vi "Ver 1.vi"() -> ()   [LabVIEW 2016]
doc: "This example VI shows how to use thermocouples to take a temperature measurement.\n\nNote:\nFor front panel measurements, make sure the Input switch is in the out position(F)\nFor plug-in card measurements, make sure the Input switch is in the in poisition(R)"
uses:
  Documents/keithley_27xx/Keithley 27XX/Public/Configure/Measurement Specific/Configure FRTD.vi
  Documents/keithley_27xx/Keithley 27XX/Public/Configure/Measurement Specific/Configure Thermocouple.vi
  Documents/keithley_27xx/Keithley 27XX/Public/Configure/Measurement Specific/Configure Thermistor.vi
  Documents/keithley_27xx/Keithley 27XX/Public/Data/Read Multiple Direct.vi
  Documents/keithley_27xx/Keithley 27XX/Keithley 27XX.lvlib
  Documents/keithley_27xx/Keithley 27XX/Public/Close.vi
panel:
  in  "Sample Size":dbl
  in  "Sensor Type":string(combo)
  in  "Delta3":dbl=1.0
  in  "Beta3":dbl=0.1
  in  "Alpha3":dbl=0.0038
  in  "Delta2":dbl=1.0
  in  "Beta2":dbl=0.1
  in  "Alpha2":dbl=0.0038
  in  "Delta1":dbl=1.0
  in  "Beta1":dbl=0.1
  in  "Alpha1":dbl=0.0038
  in  "Serial Configuration":T1={"Baud Rate (9600)"=9600, "Flow Control (1: XON/XOFF)"=1, "Termination Char (0:CR)"=0} {"Termination Char (0:CR)" items=["CR", "LF", "CRLF (Do not use)", "LFCR (Do not use)"]; "Flow Control (1: XON/XOFF)" items=["None", "XON/XOFF", "RTS/CTS (2701 Only)", "XON/XOFF & RTS/CTS (2701 Only)"]; "Baud Rate (9600)" items=["300"=300, "600"=600, "1200"=1200, "2400"=2400, "4800"=4800, "9600"=9600, "19.2k"=19200, "38.4k (2701 Only)"=38400, "57.6k (2701 Only)"=57600, "115.2k (2701 Only)"=115200]}
  in  "VISA resource name":refnum<visa-resource-name>="TCPIP0::192.168.69.200::1394::SOCKET"
  out "Output3":dbl[](array[numeric])
  in  "Channel (101) 3":string="117"
  out "Output2":dbl[](array[numeric])
  in  "Channel (101) 2":string="114"
  in  "stop":bool
  out "Output1":dbl[](array[numeric])
  in  "Channel (101)":string="113"
  in  "Temperature (0: Celsius)":u16(ring) items=["Celsius", "Fahrenheit", "Kelvin"]
  # "*For front panel measurements, make sure the Input switch is in the out position(F)*\n  For plug-in card measurements, make sure the Input switch is in the in position(R)"
  # "© 2005 National Instruments Corporation.  ALL RIGHTS RESERVED."
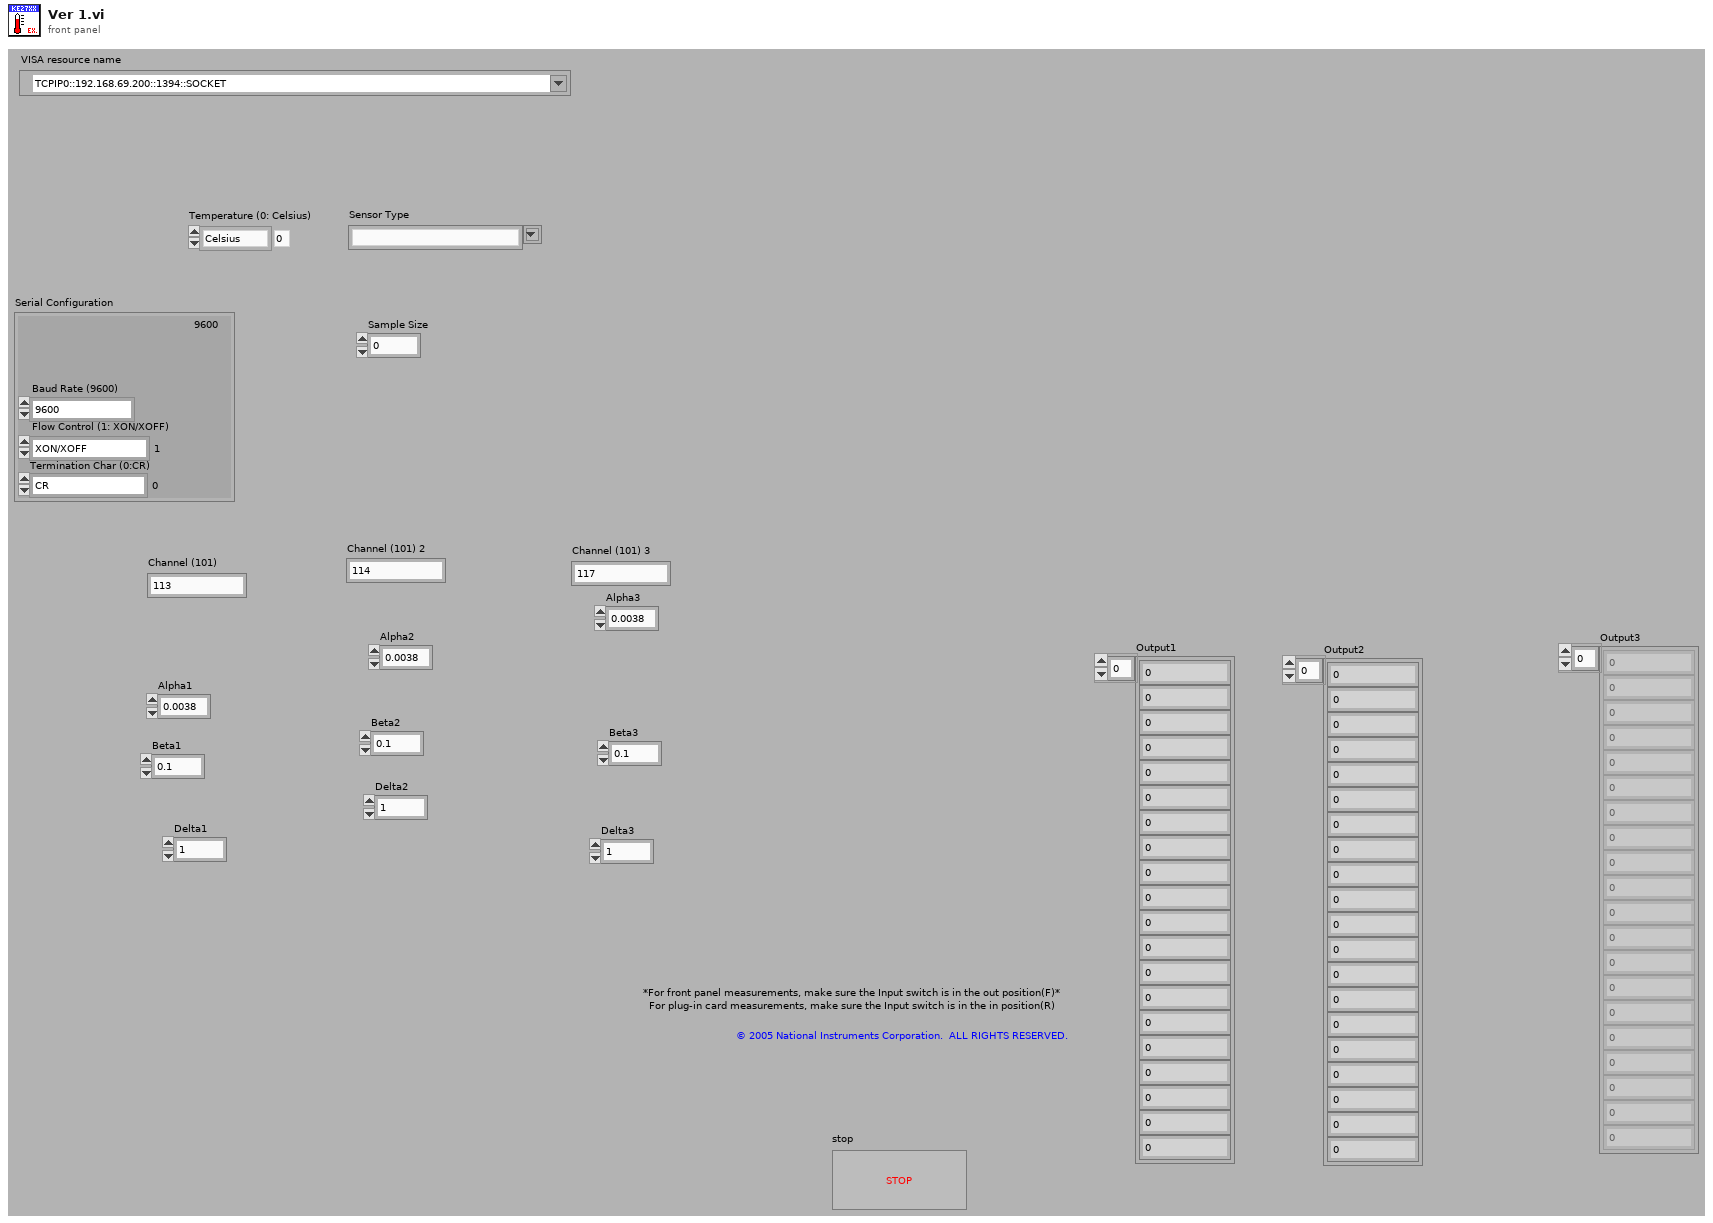
[diagram p1: front panel]
types:
  T1 = cluster{"Baud Rate (9600)":u32, "Flow Control (1: XON/XOFF)":u16, "Termination Char (0:CR)":u16}
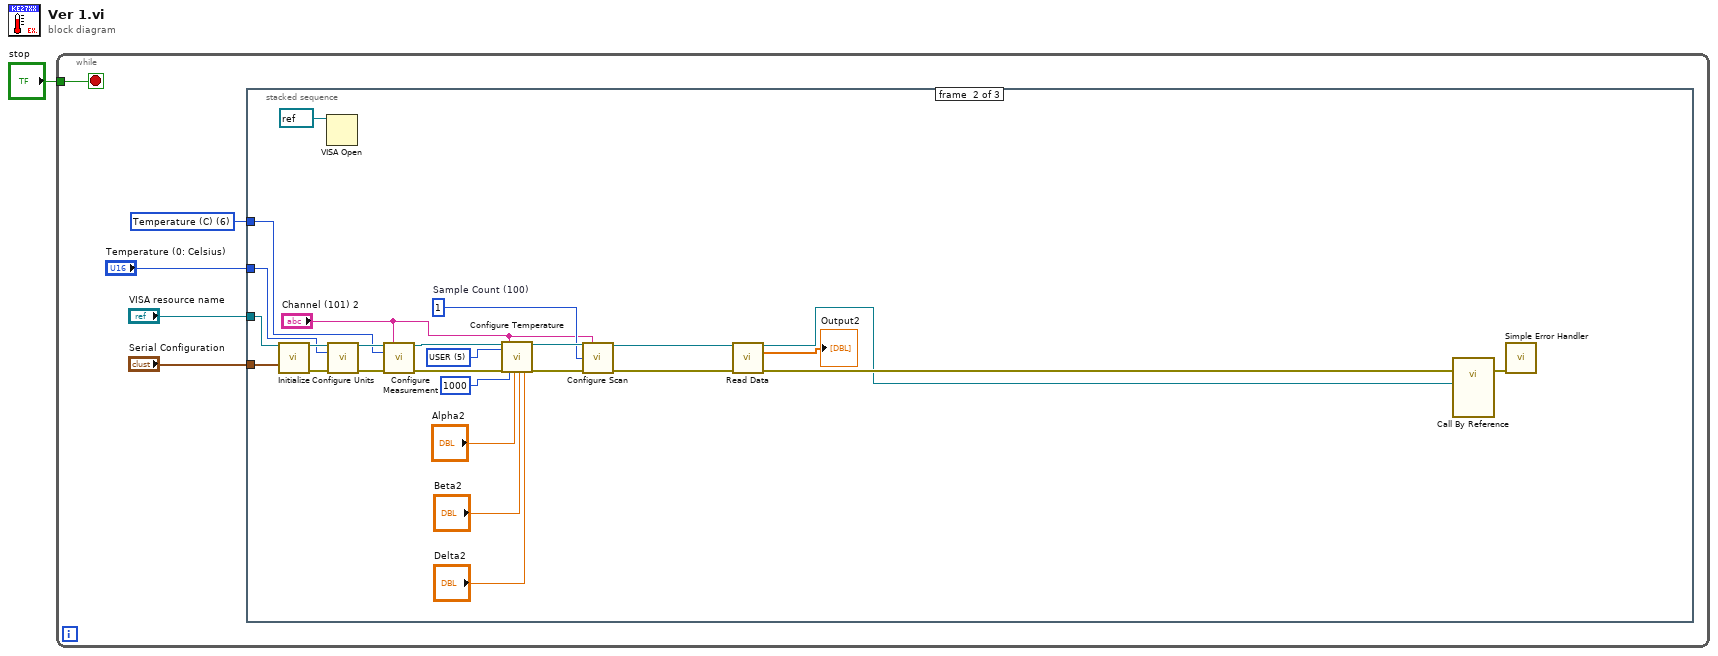
[diagram p0: block diagram]
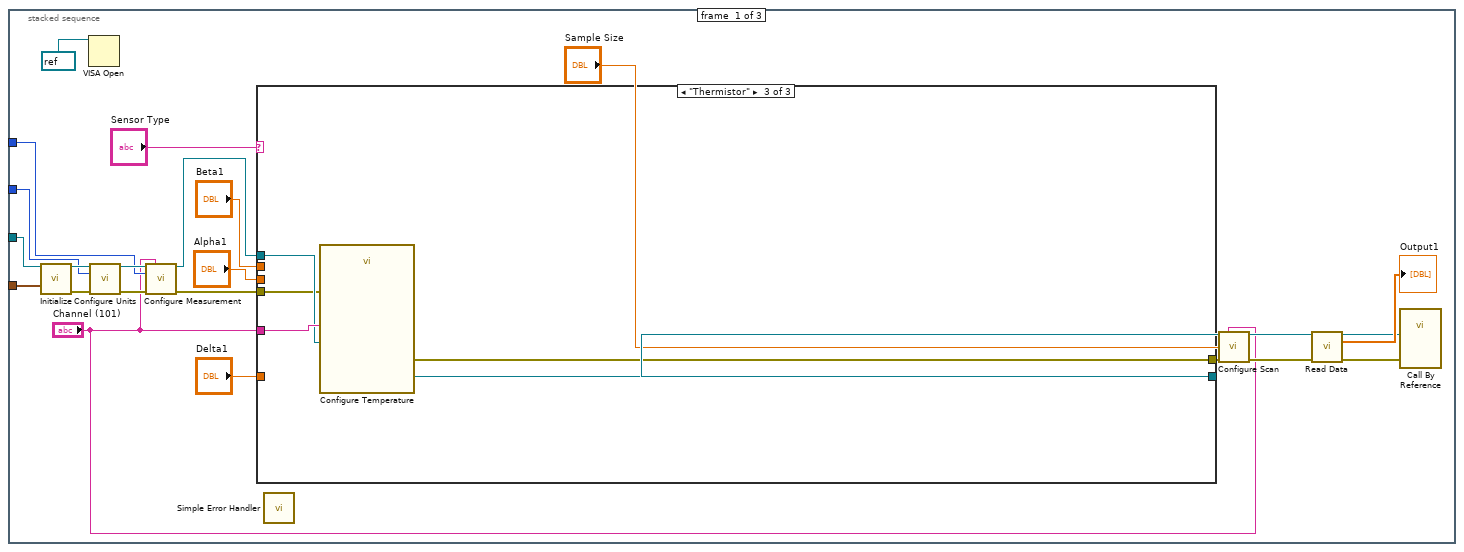
[diagram p2: hidden frame]
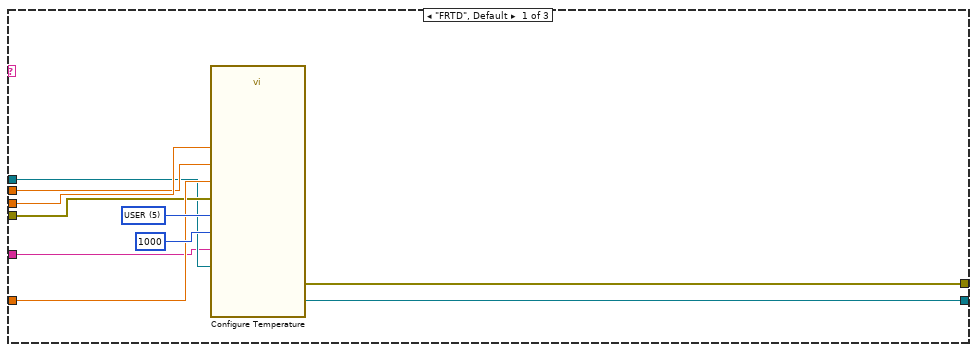
[diagram p3: hidden frame]
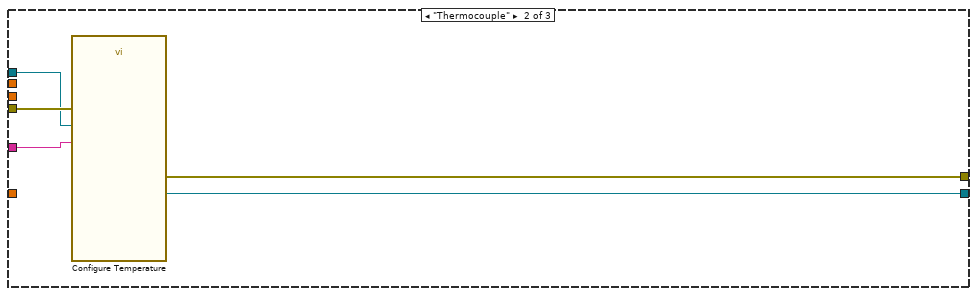
[diagram p4: hidden frame]
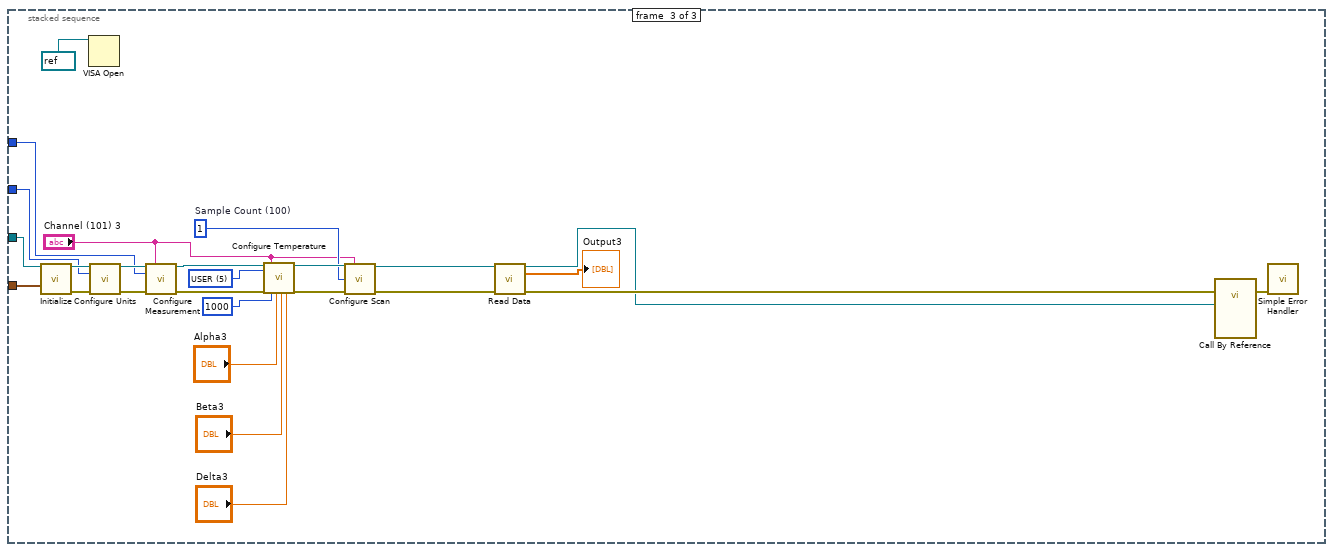
[diagram p5: hidden frame]
diagram:
  n1 = while {
    tunnel: "stop" -> [w2]
    stop <- w2 stop-if-true
    w4 = u16 6 items=["DC Voltage", "AC Voltage", "DC Current", "AC Current", "Resistance", "Four-Wire Resistance", "Temperature (C)", "Frequency", "Period", "Continuity"] ("Function (0: DC Voltage)")
    n2 = stacked-sequence {
      tunnel: "VISA resource name" -> [w22 w57 w84]
      tunnel: "Serial Configuration" -> [w21 w58 w83]
      tunnel: w4 -> [w20 w53 w79]
      tunnel: "Temperature (0: Celsius)" -> [w19 w52 w78]
      frame #0 {
        n3 = call "Initialize.vi"("VISA resource name"=w22, "Serial Configuration"=w21) -> ("VISA resource name out"=w29:refnum<visa-resource-name>, "error out"=w26:errorcluster)  [unwired: 12 in]
        n4 = VISA Open(VISA resource name=refnum<visa-resource-name> refnum) -> ()  [unwired: 4 in, 2 out]
        n5 = call "Configure Units.vi"("VISA resource name"=w29, "Temperature (0: Celsius)"=w19, "error in (no error)"=w26) -> ("VISA resource name out"=w30:refnum<visa-resource-name>, "error out"=w25:errorcluster)  [unwired: 11 in]
        n6 = call "Configure Measurement.vi"("VISA resource name"=w30, "Scan List (Empty)"="Channel (101)", "Function (0: DC Voltage)"=w20, "error in (no error)"=w25) -> ("VISA resource name out"=w12:refnum<visa-resource-name>, "error out"=w13:errorcluster)  [unwired: 10 in]
        n7 = case shown="\"Thermistor\"" "Sensor Type" {
          tunnel: [w39 w44 w50] -> w18
          tunnel: [w40 w45 w49] -> w17
          tunnel: "Delta1" -> [w34 _ _]
          tunnel: "Beta1" -> [w35 _ _]
          tunnel: "Alpha1" -> [w36 _ _]
          tunnel: w13 -> [w33 w43 w46]
          tunnel: w12 -> [w32 w42 w47]
          tunnel: "Channel (101)" -> [w31 w41 w48]
          frame "FRTD", Default {
            w38 = u16 5 items=["PT100", "D100", "F100", "PT3916", "PT385", "USER"] ("FRTD Type (0: PT100)")
            n8 = call-poly "Configure Temperature.vi"("VISA resource name"=w32, "FRTD Type (0: PT100)"=w38, "error in (no error)"=w33, "Scan List (Empty)"=w31, "R Zero (100)"=1000, "Alpha (0.00385)"=w36, "Beta (0.111)"=w35, "Delta (1.507)"=w34) -> ("VISA resource name out"=w40:refnum<visa-resource-name>, "error out"=w39:errorcluster)  [unwired: 10 in]
          }
          frame "Thermocouple" {
            n9 = call-poly "Configure Temperature.vi"("VISA resource name"=w42, "error in (no error)"=w43, "Scan List (Empty)"=w41) -> ("VISA resource name out"=w45:refnum<visa-resource-name>, "error out"=w44:errorcluster)  [unwired: 15 in]
          }
          frame "Thermistor" {
            n10 = call-poly "Configure Temperature.vi"("VISA resource name"=w47, "error in (no error)"=w46, "Scan List (Empty)"=w48) -> ("VISA resource name out"=w49:refnum<visa-resource-name>, "error out"=w50:errorcluster)  [unwired: 15 in]
          }
        }
        n11 = call <vilib>:"Simple Error Handler.vi"() -> ()  [unwired: 5 in, 5 out]
        n12 = call "Configure Scan.vi"("VISA resource name"=w17, "Channel List (101:110)"="Channel (101)", "Sample Count (100)"="Sample Size", "error in (no error)"=w18) -> ("VISA resource name out"=w27:refnum<visa-resource-name>, "error out"=w28:errorcluster)  [unwired: 10 in]
        n13 = call-poly "Read Data.vi"("VISA resource name"=w27, "error in (no error)"=w28) -> ("VISA resource name out"=w7:refnum<visa-resource-name>, "Measurement Data"=→"Output1":dbl[], "error out"=w8:errorcluster)  [unwired: 8 in, 3 out]
        n14 = call-by-ref "?"("VISA resource name"=w7, "error in (no error)"=w8) -> ()  [unwired: 15 in, 3 out]
      }
      frame #1 {
        w62 = u16 5 items=["PT100", "D100", "F100", "PT3916", "PT385", "USER"] ("FRTD Type (0: PT100)")
        w64 = 1  # Sample Count (100)
        n15 = call "Initialize.vi"("VISA resource name"=w57, "Serial Configuration"=w58) -> ("VISA resource name out"=w74:refnum<visa-resource-name>, "error out"=w67:errorcluster)  [unwired: 12 in]
        n16 = VISA Open(VISA resource name=refnum<visa-resource-name> refnum) -> ()  [unwired: 4 in, 2 out]
        n17 = call "Configure Units.vi"("VISA resource name"=w74, "Temperature (0: Celsius)"=w52, "error in (no error)"=w67) -> ("VISA resource name out"=w75:refnum<visa-resource-name>, "error out"=w66:errorcluster)  [unwired: 11 in]
        n18 = call "Configure Measurement.vi"("VISA resource name"=w75, "Scan List (Empty)"="Channel (101) 2", "Function (0: DC Voltage)"=w53, "error in (no error)"=w66) -> ("VISA resource name out"=w65:refnum<visa-resource-name>, "error out"=w76:errorcluster)  [unwired: 10 in]
        n19 = call-poly "Configure Temperature.vi"("VISA resource name"=w65, "FRTD Type (0: PT100)"=w62, "error in (no error)"=w76, "Scan List (Empty)"="Channel (101) 2", "R Zero (100)"=1000, "Alpha (0.00385)"="Alpha2", "Beta (0.111)"="Beta2", "Delta (1.507)"="Delta2") -> ("VISA resource name out"=w72:refnum<visa-resource-name>, "error out"=w71:errorcluster)  [unwired: 10 in]
        n20 = call "Configure Scan.vi"("VISA resource name"=w72, "Channel List (101:110)"="Channel (101) 2", "Sample Count (100)"=w64, "error in (no error)"=w71) -> ("VISA resource name out"=w69:refnum<visa-resource-name>, "error out"=w70:errorcluster)  [unwired: 10 in]
        n21 = call-poly "Read Data.vi"("VISA resource name"=w69, "error in (no error)"=w70) -> ("VISA resource name out"=w51:refnum<visa-resource-name>, "Measurement Data"=→"Output2":dbl[], "error out"=w68:errorcluster)  [unwired: 8 in, 3 out]
        n22 = call-by-ref "?"(error in=w68, "VISA resource name"=w51) -> (error out=w73:errorcluster)  [unwired: 15 in, 2 out]
        n23 = call <vilib>:"Simple Error Handler.vi"("error in (no error)"=w73) -> ()  [unwired: 4 in, 5 out]
      }
      frame #2 {
        w88 = u16 5 items=["PT100", "D100", "F100", "PT3916", "PT385", "USER"] ("FRTD Type (0: PT100)")
        w90 = 1  # Sample Count (100)
        n24 = call "Initialize.vi"("VISA resource name"=w84, "Serial Configuration"=w83) -> ("VISA resource name out"=w100:refnum<visa-resource-name>, "error out"=w93:errorcluster)  [unwired: 12 in]
        n25 = VISA Open(VISA resource name=refnum<visa-resource-name> refnum) -> ()  [unwired: 4 in, 2 out]
        n26 = call "Configure Units.vi"("VISA resource name"=w100, "Temperature (0: Celsius)"=w78, "error in (no error)"=w93) -> ("VISA resource name out"=w101:refnum<visa-resource-name>, "error out"=w92:errorcluster)  [unwired: 11 in]
        n27 = call "Configure Measurement.vi"("VISA resource name"=w101, "Scan List (Empty)"="Channel (101) 3", "Function (0: DC Voltage)"=w79, "error in (no error)"=w92) -> ("VISA resource name out"=w91:refnum<visa-resource-name>, "error out"=w102:errorcluster)  [unwired: 10 in]
        n28 = call-poly "Configure Temperature.vi"("VISA resource name"=w91, "FRTD Type (0: PT100)"=w88, "error in (no error)"=w102, "Scan List (Empty)"="Channel (101) 3", "R Zero (100)"=1000, "Alpha (0.00385)"="Alpha3", "Beta (0.111)"="Beta3", "Delta (1.507)"="Delta3") -> ("VISA resource name out"=w98:refnum<visa-resource-name>, "error out"=w97:errorcluster)  [unwired: 10 in]
        n29 = call "Configure Scan.vi"("VISA resource name"=w98, "Channel List (101:110)"="Channel (101) 3", "Sample Count (100)"=w90, "error in (no error)"=w97) -> ("VISA resource name out"=w95:refnum<visa-resource-name>, "error out"=w96:errorcluster)  [unwired: 10 in]
        n30 = call-poly "Read Data.vi"("VISA resource name"=w95, "error in (no error)"=w96) -> ("VISA resource name out"=w77:refnum<visa-resource-name>, "Measurement Data"=→"Output3":dbl[], "error out"=w94:errorcluster)  [unwired: 8 in, 3 out]
        n31 = call-by-ref "?"(error in=w94, "VISA resource name"=w77) -> (error out=w99:errorcluster)  [unwired: 15 in, 2 out]
        n32 = call <vilib>:"Simple Error Handler.vi"("error in (no error)"=w99) -> ()  [unwired: 4 in, 5 out]
      }
    }
  }
